vi "Write_ToScreensEvent.vi"(8 "error in (no error)":errorcluster, 10 "To Screens Event":refnum<user-event>, 11 "EVE in":refnum<class "EVE.lvclass">) -> (0 "error out":errorcluster, 3 "EVE out":refnum<class "EVE.lvclass">)   [LabVIEW 2013, in "EVE.lvclass"]
uses:
  EVE.lvclass
  030 - EVENTS/02 - ToScreens/ToScreen.ctl
  030 - EVENTS/02 - ToScreens/ToScreensCommand.ctl
  EVE.lvclass/EVE.ctl
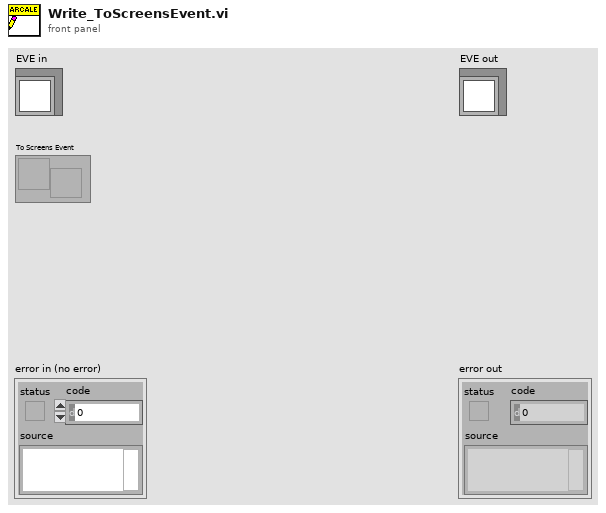
[diagram p1: front panel]
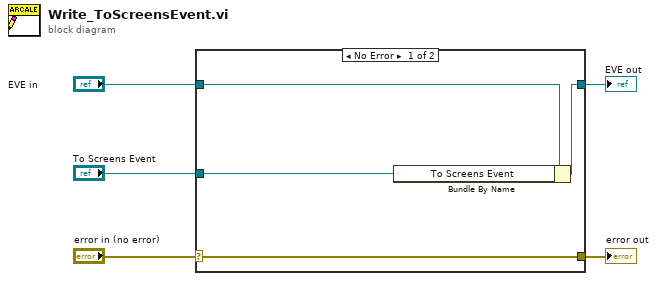
[diagram p0: block diagram]
diagram:
  n1 = case shown="No Error" "error in (no error)" {
    selector: "error in (no error)" -> [w9 w10]
    tunnel: [w9 w10] -> w4
    tunnel: [w7 w11] -> w2
    tunnel: "EVE in" -> [w8 w11]
    tunnel: "To Screens Event" -> [w6 _]
    frame No Error {
      n2 = Bundle By Name(cluster=w8, "To Screens Event"=w6) -> (w7:refnum<class "EVE.lvclass">)
    }
    frame Error {
    }
  }
  "error out" <- w4
  "EVE out" <- w2
